vi "test Default Use is Case Sensitive.vi"(8 "error in (no error)":errorcluster, 11 "TestCase in":refnum<class "Pass If Equal 1D Array (String) Test Case.lvclass">) -> (0 "error out":errorcluster, 3 "TestCase out":refnum<class "Pass If Equal 1D Array (String) Test Case.lvclass">)   [LabVIEW 2015, in "Pass If Equal 1D Array (String) Test Case.lvclass"]
uses:
  Pass If Equal 1D Array (String) Test Case.lvclass
  <vilib>/addons/_JKI Toolkits/VI Tester/TestCase.llb/TestCase.lvclass
  VITAC.lvlib
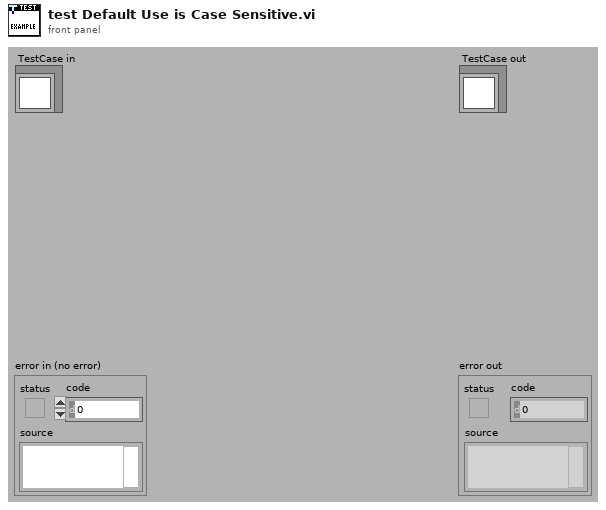
[diagram p1: front panel]
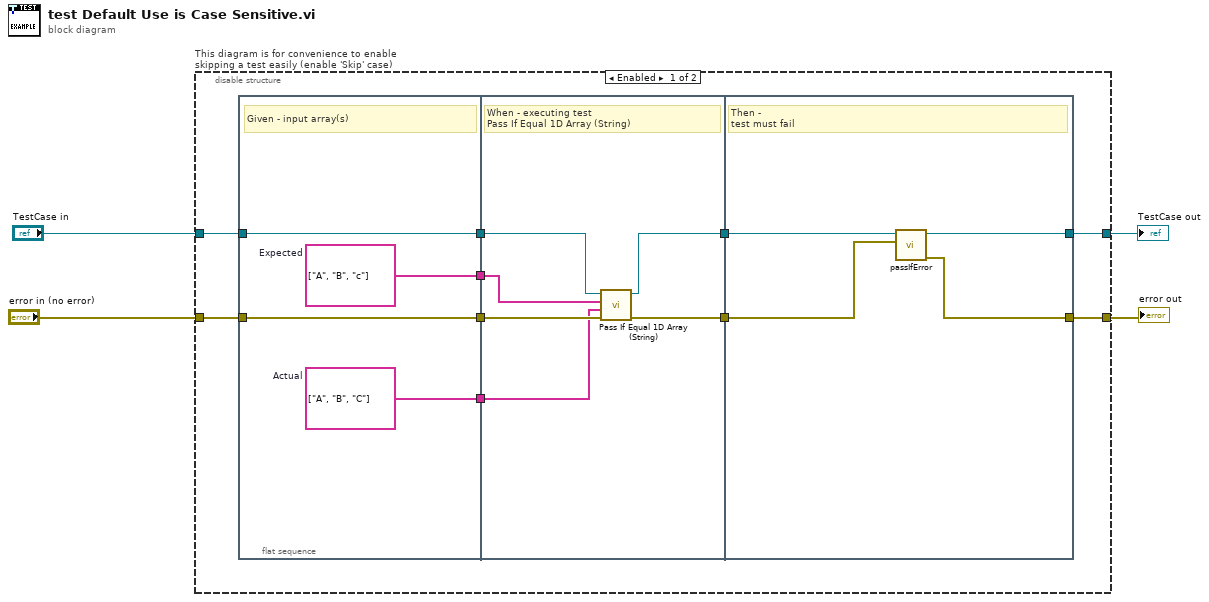
[diagram p0: block diagram]
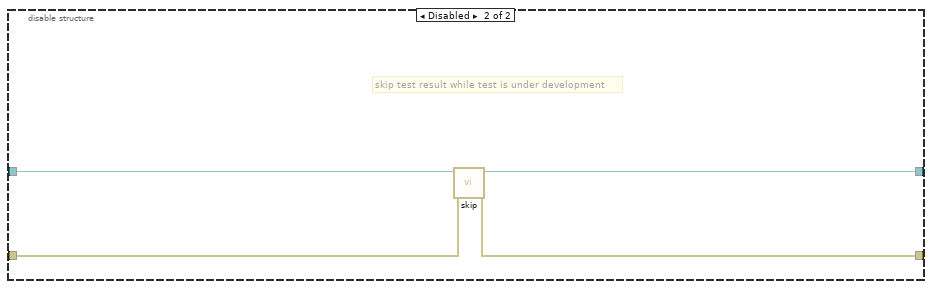
[diagram p2: hidden frame]
diagram:
  n1 = disable-structure "This diagram is for convenience to enable skipping a test easily (enable 'Skip' case)" shown="Enabled" {
    disable-tunnel: "TestCase in" -> [w11 w32]
    disable-tunnel: [w14 w30] -> w1
    disable-tunnel: [w10 w31] -> w3
    disable-tunnel: "error in (no error)" -> [w7 w29]
    frame Enabled {
      n2 = flat-sequence {
        tunnel: [w18] -> w12
        tunnel: w11 -> [w18]
        tunnel: [w17] -> w8
        tunnel: w7 -> [w17]
        tunnel: [w16] -> w6
        tunnel: [w15] -> w5
        tunnel: [w21] -> w13
        tunnel: w12 -> [w22]
        tunnel: [w23] -> w9
        tunnel: w8 -> [w24]
        tunnel: w6 -> [w20]
        tunnel: w5 -> [w19]
        tunnel: [w25] -> w14
        tunnel: w13 -> [w26]
        tunnel: [w27] -> w10
        tunnel: w9 -> [w28]
        frame #0 {
          w16 = string[] ["A", "B", "C"]  # Actual
          w15 = string[] ["A", "B", "c"]  # Expected
          # "Given - input array(s)"
        }
        frame #1 {
          # "When - executing test \nPass If Equal 1D Array (String)"
          n3 = call "Pass If Equal 1D Array (String).vi"("error in (no error)"=w24, "actual"=w20, "expected"=w19, "TestCase in"=w22) -> ("error out"=w23:errorcluster, "TestCase out"=w21:refnum<class "Pass If Equal 1D Array (String) Test Case.lvclass">)  [unwired: 6 in]
        }
        frame #2 {
          # "Then - \ntest must fail"
          n4 = call-dynamic "passIfError.vi"("error"=w28, "TestCase in"=w26) -> ("error out"=w27:errorcluster, "TestCase out"=w25:refnum<class "Pass If Equal 1D Array (String) Test Case.lvclass">)  [unwired: 8 in]
        }
      }
    }
    frame Disabled {
      # "skip test result while test is under development"
      n5 = call <vilib>:"skip.vi"("error in (no error)"=w29, "TestCase in"=w32) -> ("error out"=w31:errorcluster, "TestCase out"=w30:refnum<class "Pass If Equal 1D Array (String) Test Case.lvclass">)  [unwired: 8 in]
    }
  }
  "error out" <- w3
  "TestCase out" <- w1
